vi "MTM2_getSample_tangentActuatorPositionAbsoluteEncoderPositionMeasured.vi"(8 "error in (no error)":errorcluster, 11 "tangentActuatorPositionAbsoluteEncoderPositionMeasured_Ctl":T1) -> (0 "error out":errorcluster, 2 "function return":i32, 3 "tangentActuatorPositionAbsoluteEncoderPositionMeasured_Ctl out":T1)   [LabVIEW 2018, in "SALLV_MTM2.lvlib"]
doc: "int MTM2_shm_getSample_tangentActuatorPositionAbsoluteEncoderPositionMeasuredLV(MTM2_tangentActuatorPositionAbsoluteEncoderPositionMeasuredLV *tangentActuatorPositionAbsoluteEncoderPositionMeasured_Ctl );"
uses:
  SALLV_MTM2.lvlib
  DataTypes/tangentActuatorPositionAbsoluteEncoderPositionMeasured.ctl
  SALLV_MTM2.so
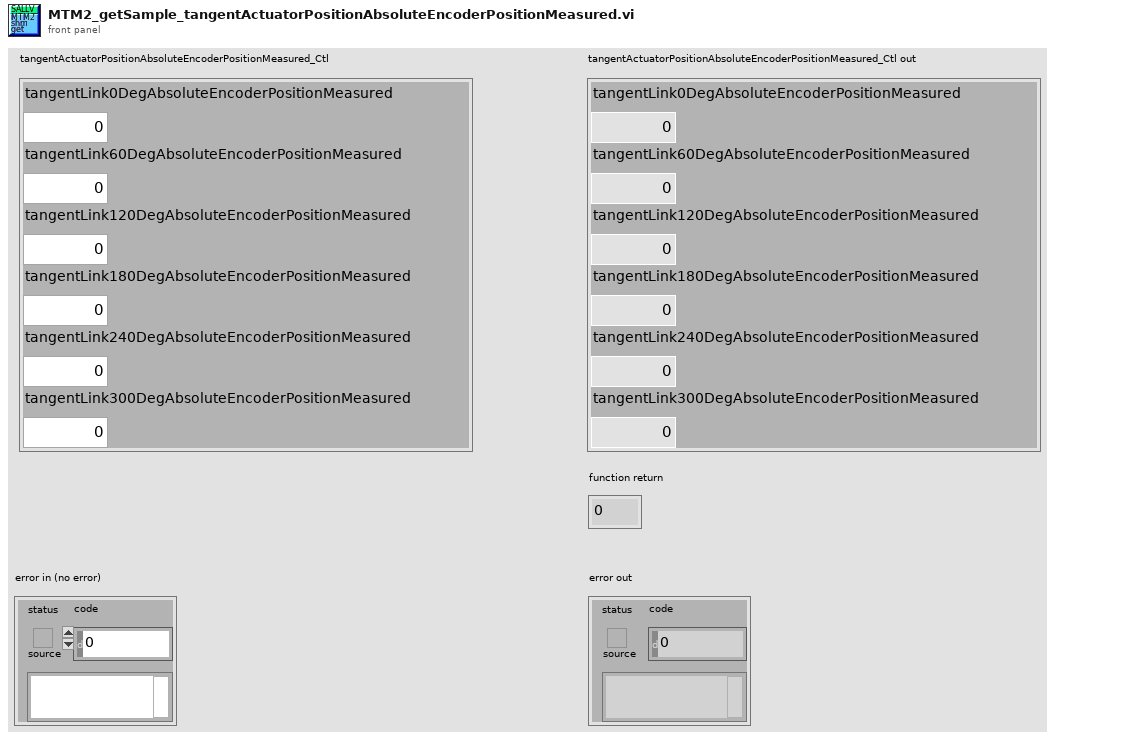
[diagram p1: front panel]
types:
  T1 = typedef "SALLV_MTM2.lvlib/tangentActuatorPositionAbsoluteEncoderPositionMeasured.ctl" = cluster{"tangentLink0DegAbsoluteEncoderPositionMeasured":dbl, "tangentLink60DegAbsoluteEncoderPositionMeasured":dbl, "tangentLink120DegAbsoluteEncoderPositionMeasured":dbl, "tangentLink180DegAbsoluteEncoderPositionMeasured":dbl, "tangentLink240DegAbsoluteEncoderPositionMeasured":dbl, "tangentLink300DegAbsoluteEncoderPositionMeasured":dbl}
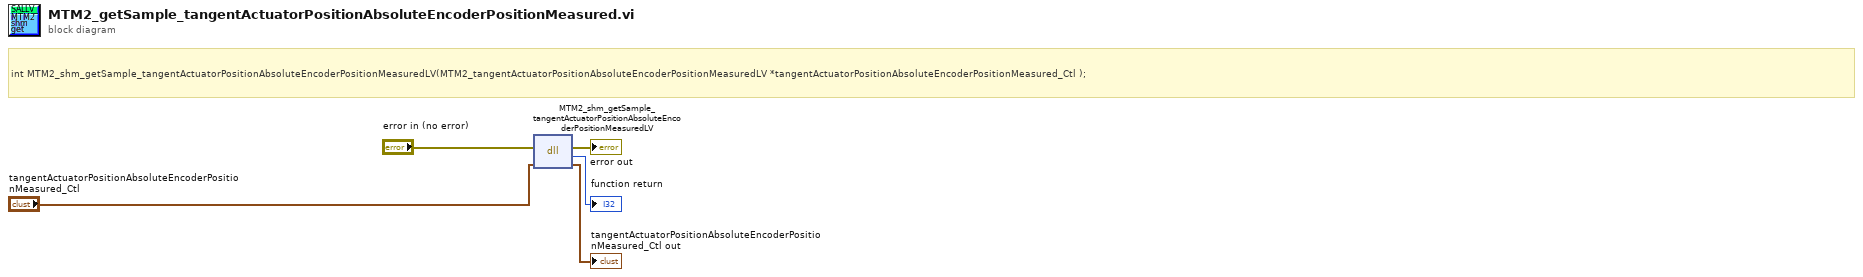
[diagram p0: block diagram]
diagram:
  # "int MTM2_shm_getSample_tangentActuatorPositionAbsoluteEncoderPositionMeasuredLV(MTM2_tangentActuatorPositionAbsoluteEncoderPositionMeasuredLV *tangentActuatorPositionAbsoluteEncoderPositionMeasured_Ctl );"
  n1 = dll-call lib="home/ttsai/Document/salApiMTM2/SALLV_MTM2/SALLV_MTM2.*" fn="MTM2_shm_getSample_tangentActuatorPositionAbsoluteEncoderPositionMeasuredLV"(error in="error in (no error)", "tangentActuatorPositionAbsoluteEncoderPositionMeasured_Ctl"="tangentActuatorPositionAbsoluteEncoderPositionMeasured_Ctl") -> (error out=→"error out":errorcluster, →"function return":i32, "tangentActuatorPositionAbsoluteEncoderPositionMeasured_Ctl"=→"tangentActuatorPositionAbsoluteEncoderPositionMeasured_Ctl out":T1)  [unwired: 2 in, 1 out]
